vi "Read Enqueuer.vi"   [LabVIEW 2020]
uses:
  <vilib>/ActorFramework/Actor/Actor.lvclass
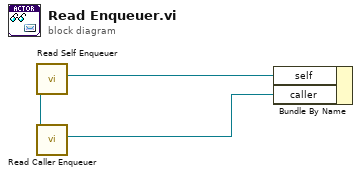
[diagram p0: block diagram]
diagram:
  n1 = call <vilib>:"Read Caller Enqueuer.vi"() -> ("Caller Enqueuer"=w2:refnum<class "Message Enqueuer.lvclass">, "Actor"=w4:refnum<class "Actor.lvclass">)  [unwired: 10 in]
  n2 = call <vilib>:"Read Self Enqueuer.vi"("Actor"=w4) -> ("Self Enqueuer"=w3:refnum<class "Message Enqueuer.lvclass">)  [unwired: 10 in]
  n3 = Bundle By Name("self"=w3, "caller"=w2) -> (w1:cluster{}, w5:cluster{})
